vi "create_all_rt_message_queues.vi"(8 "error in (no error)":errorcluster caption="错误输入（无错误）") -> (0 "error out":errorcluster caption="错误输出", 3 "Message Queues":T1 caption="消息队列")   [LabVIEW 2015, in "message_queue.lvlib"]
doc: "本VI用于创建应用程序所需的所有消息队列。如应用程序需要两个以上消息队列，可右键单击上面的“消息队列”常量并选择“打开自定义类型”，将新的消息队列添加至该自定义类型，然后通过本VI进行初始化。"
uses:
  message_queue.lvlib
  all_rt_message_queues.ctl
  message_cluster.ctl
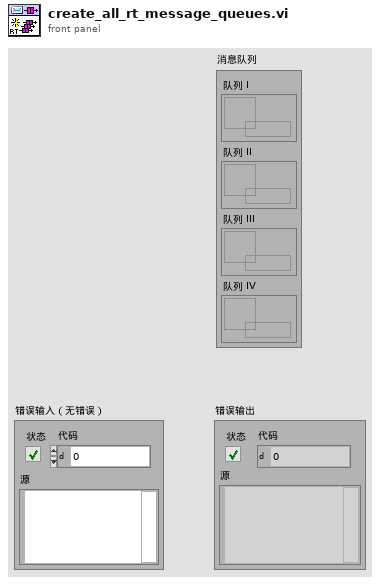
[diagram p1: front panel]
types:
  T1 = typedef "message_queue.lvlib/all_rt_message_queues.ctl" = cluster{"Queue I":refnum<queue>, "Queue II":refnum<queue>, "Queue III":refnum<queue>, "Queue IV":refnum<queue>}
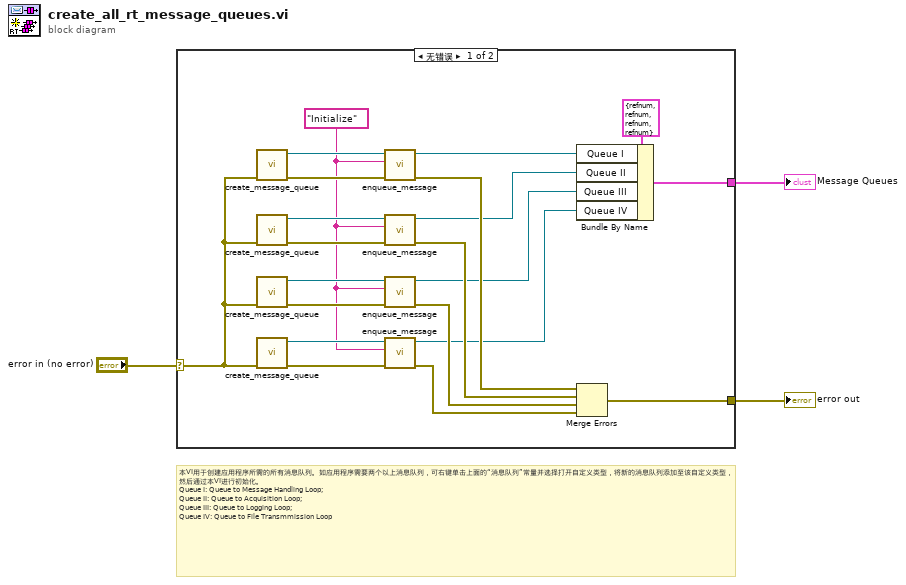
[diagram p0: block diagram]
diagram:
  # "本VI用于创建应用程序所需的所有消息队列。如应用程序需要两个以上消息队列，可右键单击上面的“消息队列”常量并选择打开自定义类型，将新的消息队列添加至该自定义类型，然后通过本VI进行初始化。 \nQueue I: Queue to Message Handling Loop;\nQueue II: Queue to Acquisition Loop; \nQueue III: Queue to Logging Loop; \nQueue IV: Queue to File Transmmission Loop"
  n1 = case shown="无错误" "error in (no error)" {
    selector: "error in (no error)" -> [w13 w25]
    tunnel: [w18 w25] -> w3
    tunnel: [w21 _] -> w1
    frame No Error {
      w7 = "Initialize" ("Message")
      n2 = call "create_message_queue.vi"("error in (no error)"=w13) -> ("error out"=w16:errorcluster, "Message Queue"=w17:refnum<queue>)  [unwired: 9 in]
      n3 = call "create_message_queue.vi"("error in (no error)"=w13) -> ("error out"=w20:errorcluster, "Message Queue"=w19:refnum<queue>)  [unwired: 9 in]
      n4 = call "create_message_queue.vi"("error in (no error)"=w13) -> ("error out"=w11:errorcluster, "Message Queue"=w12:refnum<queue>)  [unwired: 9 in]
      n5 = call "create_message_queue.vi"("error in (no error)"=w13) -> ("error out"=w6:errorcluster, "Message Queue"=w8:refnum<queue>)  [unwired: 9 in]
      n6 = call "enqueue_message.vi"("error in (no error)"=w16, "Message"=w7, "Message Queue"=w17) -> ("error out"=w24:errorcluster, "dup Message Queue"=w15:refnum<queue>)  [unwired: 7 in]
      n7 = call "enqueue_message.vi"("error in (no error)"=w20, "Message"=w7, "Message Queue"=w19) -> ("error out"=w23:errorcluster, "dup Message Queue"=w14:refnum<queue>)  [unwired: 7 in]
      n8 = call "enqueue_message.vi"("error in (no error)"=w11, "Message"=w7, "Message Queue"=w12) -> ("error out"=w9:errorcluster, "dup Message Queue"=w10:refnum<queue>)  [unwired: 7 in]
      n9 = call "enqueue_message.vi"("error in (no error)"=w6, "Message"=w7, "Message Queue"=w8) -> ("error out"=w5:errorcluster, "dup Message Queue"=w4:refnum<queue>)  [unwired: 7 in]
      n10 = Bundle By Name(cluster=T1 {"Queue I"=refnum, "Queue II"=refnum, "Queue III"=refnum, "Queue IV"=refnum} ("Message Queues"), "Queue I"=w15, "Queue II"=w14, "Queue III"=w10, "Queue IV"=w4) -> (w21:T1)
      n11 = Merge Errors(w24, w23, w9, w5) -> (w18:errorcluster)
    }
    frame Error {
    }
  }
  "error out" <- w3
  "Message Queues" <- w1
